vi "PH_gentec_P-Link.set Enable Anticipation.vi"(0 "i ref in":refnum<vi>, 2 "VISA resource in":refnum<visa-resource-name>, 5 "error in":errorcluster) -> (11 "Timeout":bool, 13 "Data read":string[](array[string]), 14 "i ref out":refnum<vi>, 16 "VISA resource out":refnum<visa-resource-name>, 17 "Error":bool, 18 "Failure":bool, 19 "error out":errorcluster)   [LabVIEW 2014, in "PH_gentec_P-Link.lvlib"]
doc: "This VI writes wanted Settings to the Device and checks the result."
uses:
  PH_gentec_P-Link.lvlib
  instr.lib/Gentec-P-Link/gentec-P-Link - Driver.lvlib
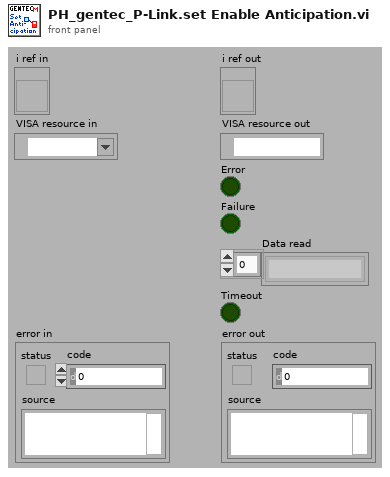
[diagram p1: front panel]
types:
  T1 = typedef "PH_gentec_P-Link.lvlib/PH_gentec_P-Link.i attribute.ctl" = cluster{"GUI References":cluster{"Wanted Head Settings":refnum<vi>, "Current Head Settings":refnum<vi>, "Set Auto Range":refnum<vi>, "Trigger Polarity":refnum<vi>, "Trigger Source":refnum<vi>, "Waveform Averages":refnum<vi>, "Continuous":refnum<vi>, "get one Value":refnum<vi>}, "Wanted Head Settings":T2, "Current Head Settings":T2}
  T2 = typedef "PH_gentec_P-Link.lvlib/PH_gentec_P-Link.Head Settings.ctl" = cluster{"Measurement Mode":T3, "Enable Anticipation":bool, "Set Auto Range":bool, "Block Signal":bool, "Set Head Attenuator":bool, "Enable SSE":bool, "Trigger Polarity":T4, "Trigger Source":T5, "Waveform Averages":T6, "Set Zero":i32, "Current Measurement":i32, "Start Data Flow":bool}
  T3 = typedef "gentec-M-Link - Driver.lvlib/gentec-M-Link.Measurement Mode.ctl" = u16
  T4 = typedef "gentec-M-Link - Driver.lvlib/gentec-M-Link.Trigger Polarity.ctl" = u16
  T5 = typedef "gentec-M-Link - Driver.lvlib/gentec-M-Link.Trigger Source.ctl" = u16
  T6 = typedef "gentec-M-Link - Driver.lvlib/gentec-M-Link.Waveform Averages.ctl" = u16
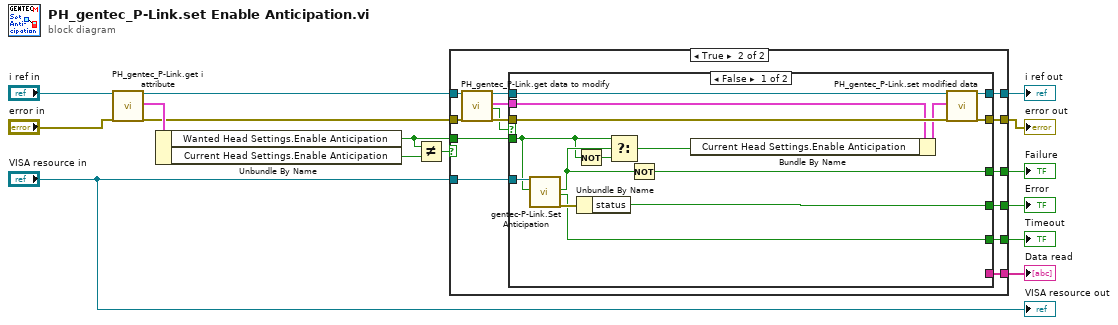
[diagram p0: block diagram]
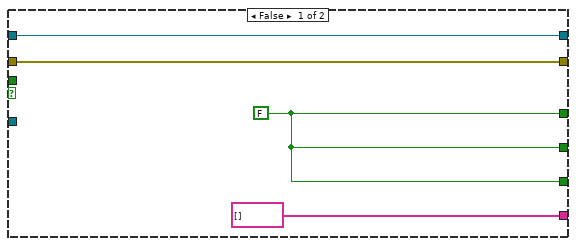
[diagram p2: hidden frame]
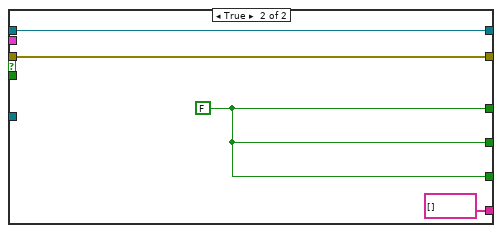
[diagram p3: hidden frame]
diagram:
  n1 = call "PH_gentec_P-Link.get i attribute.vi"("i ref in"="i ref in", "error in (no error)"="error in") -> ("i ref out"=w10:refnum<vi>, "i attribute"=w13:T1, "error out"=w12:errorcluster)  [unwired: 15 in]
  n2 = Unbundle By Name(w13) -> ("Wanted Head Settings.Enable Anticipation"=w6:bool, "Current Head Settings.Enable Anticipation"=w7:bool)
  n3 = Not Equal?(x=w6, y=w7) -> (x != y?=w5:bool)
  n4 = case shown="True" w5 {
    tunnel: [w18 w33] -> w15
    tunnel: [w19 w32] -> w14
    tunnel: w12 -> [w18 w27]
    tunnel: w10 -> [w19 w26]
    tunnel: "VISA resource in" -> [_ w25]
    tunnel: w6 -> [_ w24]
    tunnel: [w17 w23] -> w4
    tunnel: [w17 w22] -> w3
    tunnel: [w17 w21] -> w2
    tunnel: [string[] [] w20] -> w1
    frame False {
      w17 = FALSE
    }
    frame True {
      n5 = call "PH_gentec_P-Link.get data to modify.vi"("i ref in"=w26, "error in (no error)"=w27) -> ("i ref out"=w30:refnum<vi>, "i attribute"=w29:T1, "timed out"=w28:bool, "error out"=w31:errorcluster)  [unwired: 14 in]
      n6 = case shown="False" w28 {
        tunnel: w25 -> [w36 _]
        tunnel: [w45 w52] -> w32
        tunnel: [w44 w51] -> w33
        tunnel: w31 -> [w47 w51]
        tunnel: w30 -> [w48 w52]
        tunnel: w29 -> [w41 _]
        tunnel: w24 -> [w35 _]
        tunnel: [w40 w50] -> w23
        tunnel: [w39 w50] -> w22
        tunnel: [w34 w50] -> w21
        tunnel: [_ string[] []] -> w20
        frame False {
          n7 = call "gentec-P-Link.Set Anticipation.vi"("VISA resource name"=w36, "On/Off"=w35) -> ("Sucess?"=w38:bool, "TimeOut?"=w34:bool, "error out"=w37:errorcluster)  [unwired: 14 in, 1 out]
          n8 = Not(x=w35) -> (.not. x?=w43:bool)
          n9 = Unbundle By Name(w37) -> ("status"=w40:bool)
          n10 = Select(t=w35, s=w38, f=w43) -> (s? t:f=w42:bool)
          n11 = Not(x=w38) -> (.not. x?=w39:bool)
          n12 = Bundle By Name(cluster=w41, "Current Head Settings.Enable Anticipation"=w42) -> (w46:T1)
          n13 = call "PH_gentec_P-Link.set modified data.vi"("i ref in"=w48, "i attribute"=w46, "error in (no error)"=w47) -> ("i ref out"=w45:refnum<vi>, "error out"=w44:errorcluster)  [unwired: 15 in]
        }
        frame True {
          w50 = FALSE
        }
      }
    }
  }
  "error out" <- w15
  "i ref out" <- w14
  "Data read" <- w1
  "Timeout" <- w2
  "Error" <- w4
  "Failure" <- w3
  "VISA resource out" <- "VISA resource in"
